vi "macro_MatBuilder_Fill.vi"   [LabVIEW 2019, in "Trajectory_Library.lvlib"]
uses:
  MatBuilder_Create.vi
  Trajectory_Library.lvlib
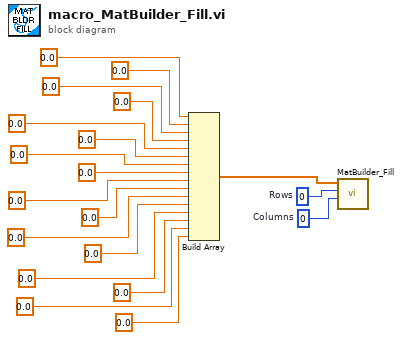
[diagram p0: block diagram]
diagram:
  w18 = 0  # Columns
  w19 = 0  # Rows
  n1 = Build Array(0.0 ("element"), 0.0 ("element"), 0.0 ("element"), 0.0 ("element"), 0.0 ("element"), 0.0 ("element"), 0.0 ("element"), 0.0 ("element"), 0.0 ("element"), 0.0 ("element"), 0.0 ("element"), 0.0 ("element"), 0.0 ("element"), 0.0 ("element"), 0.0 ("element"), 0.0 ("element")) -> (w1:dbl[])
  n2 = call "MatBuilder_Fill.vi"("Columns"=w18, "Rows"=w19, "Value List"=w1) -> ()  [unwired: 8 in, 1 out]
